vi "Main.vi"(11 "Module Admin":refnum<class "Delacor_lib_QMH_Module Admin.lvclass">) -> ()   [LabVIEW 2024, in "DQMH Power Requests.lvlib"]
doc: "This template is based off of the Queued Message Handler design pattern and the Queued Message Handler project template that ships with LabVIEW.\n\nThe main difference is that the queue is private to this module and communication between modules is performed via Broadcast and Request events.\n\nRequest events are wrapped in public API methods and are handled in the Event Handling Loop (EHL) of this VI. Any module can register for Broadcast events sent by this module. The EHL generates messages based on user interface actions.\n\nThe Message Handling Loop (MHL) processes messages generated by the EHL, or by other messages. The messages are string values, so new messages can be added easily to the Message Cases case structure in the MHL. Each message cluster can also provide an optional value for Message Data, which is a variant that can be converted to whatever message-specific data is required.\n_____\nBased on Delacor QMH Project Template 4.2.1.64.\n\n<b>Note:</b> This VI was modified by the <b>Validate DQMH Module</b> tool to have the module name be passed as the Additional Information parameter with an Error Reported broadcast.\n\n<b>Note:</b> This VI was modified by the <b>Validate DQMH Module</b> tool to call the Release Message Queue VI in the top-level Error case.\n\n<b>Note:</b> This VI was modified by the <b>Validate DQMH Module</b> tool to add a 'Panel Hidden' status updated broadcast to the Panel Close? event when External Launch = TRUE.\n\n<b>Note:</b> This VI was modified by the <b>Validate DQMH Module</b> tool to add a call to the Error Reported VI at the end of the 'Exit' MHL frame."
uses:
  DQMH Power Requests.lvlib
  <vilib>/Delacor/Delacor QMH/Libraries/Module Admin_class/Delacor_lib_QMH_Module Admin.lvclass
  Module Data--cluster.ctl
  <vilib>/Delacor/Delacor QMH/Libraries/Message Queue_class/Delacor_lib_QMH_Message Queue.lvclass/Delacor_lib_QMH_Message Queue.ctl
  Stop Argument--cluster.ctl
  <vilib>/Delacor/Delacor QMH/Libraries/Module Admin_class/Delacor_lib_QMH_Module Admin.lvclass/Delacor_lib_QMH_Module Admin.ctl
  Create Request Argument--cluster.ctl
  Create Request (Reply Payload)--cluster.ctl
  System Required Argument--cluster.ctl
  System Required (Reply Payload)--cluster.ctl
  Display Required Argument--cluster.ctl
  Display Required (Reply Payload)--cluster.ctl
  <vilib>/Utility/miscctls.llb/LVPointTypeDef.ctl
  <vilib>/Delacor/Delacor QMH/Libraries/Message Queue_class/Delacor_lib_QMH_Enqueue Message (Single).vi
  <vilib>/Delacor/Delacor QMH/Libraries/Module Admin_class/Delacor_lib_QMH_Get External Launch.vi
  <vilib>/Utility/error.llb/Error Cluster From Error Code.vi
  <vilib>/ErrorRing/Error Ring.xnode
  <vilib>/Delacor/Delacor QMH/Libraries/Message Queue_class/Delacor_lib_QMH_Message Queue.lvclass
panel:
  in  "Simulate MHL Error":bool
  in  "Simulate EHL Error":bool
  out "error out":errorcluster
  out "Status":string
  # "Other QMH Modules communicate with this Module via its Public API (wrappers for its Request Events).\n\nThis Module communicates with other Modules via its Broadcast Events.\nAny module that wants to get these messages, just registers for this module's Broadcast events."
  # "This template is for the Delacor Modified Queued Message Handler design pattern.\n\nSee the block diagram for more information on how to use this template."
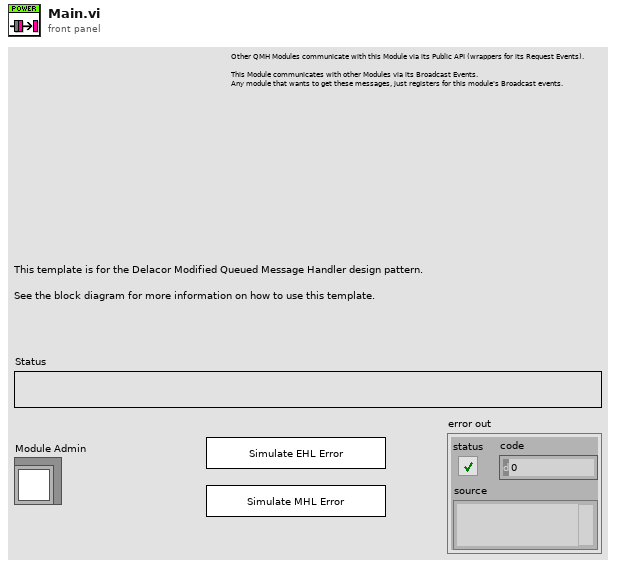
[diagram p1: front panel]
types:
  T1 = typedef "DQMH Power Requests.lvlib/Request Events--cluster.ctl" = cluster{"Stop Module":refnum<user-event>, "Show Panel":refnum<user-event>, "Hide Panel":refnum<user-event>, "Get Module Execution Status":refnum<user-event>, "Show Diagram":refnum<user-event>, "Create Request":refnum<user-event>, "System Required":refnum<user-event>, "Display Required":refnum<user-event>}
  T2 = typedef "DQMH Power Requests.lvlib/Module Data--cluster.ctl" = cluster{"Status":string, "Request Created":bool, "System Required":bool, "Display Required":bool}
  T3 = enum32{"invalid lock state", "Not Locked", "Locked (No Password)", "Password-protected"}
  T4 = typedef "DQMH Power Requests.lvlib/Stop Argument--cluster.ctl" = cluster{"Origin":string, "Exit via Stop Module Req?":bool, "Wait for Module to stop?":bool}
  T5 = typedef "DQMH Power Requests.lvlib/Create Request Argument--cluster.ctl" = cluster{"Simple Reason String":string, "Create":bool, "Wait Notifier":refnum<notifier>, "wait for reply":bool}
  T6 = typedef "DQMH Power Requests.lvlib/System Required Argument--cluster.ctl" = cluster{"Create":bool, "Wait Notifier":refnum<notifier>, "wait for reply":bool}
  T7 = typedef "DQMH Power Requests.lvlib/Display Required Argument--cluster.ctl" = cluster{"Create":bool, "Wait Notifier":refnum<notifier>, "wait for reply":bool}
  T8 = typedef "LVPointTypeDef.ctl" = cluster{"Horizontal":i16, "Vertical":i16}
  T9 = enum32{"Invalid", "Standard", "Closed", "Hidden", "Minimized", "Maximized"}
  T10 = typedef "DQMH Power Requests.lvlib/Create Request (Reply Payload)--cluster.ctl" = cluster{"Successful":bool, "Create Request_error":errorcluster}
  T11 = typedef "DQMH Power Requests.lvlib/System Required (Reply Payload)--cluster.ctl" = cluster{"Successful":bool, "System Required_error":errorcluster}
  T12 = typedef "DQMH Power Requests.lvlib/Display Required (Reply Payload)--cluster.ctl" = cluster{"Successful":bool, "Display Required_error":errorcluster}
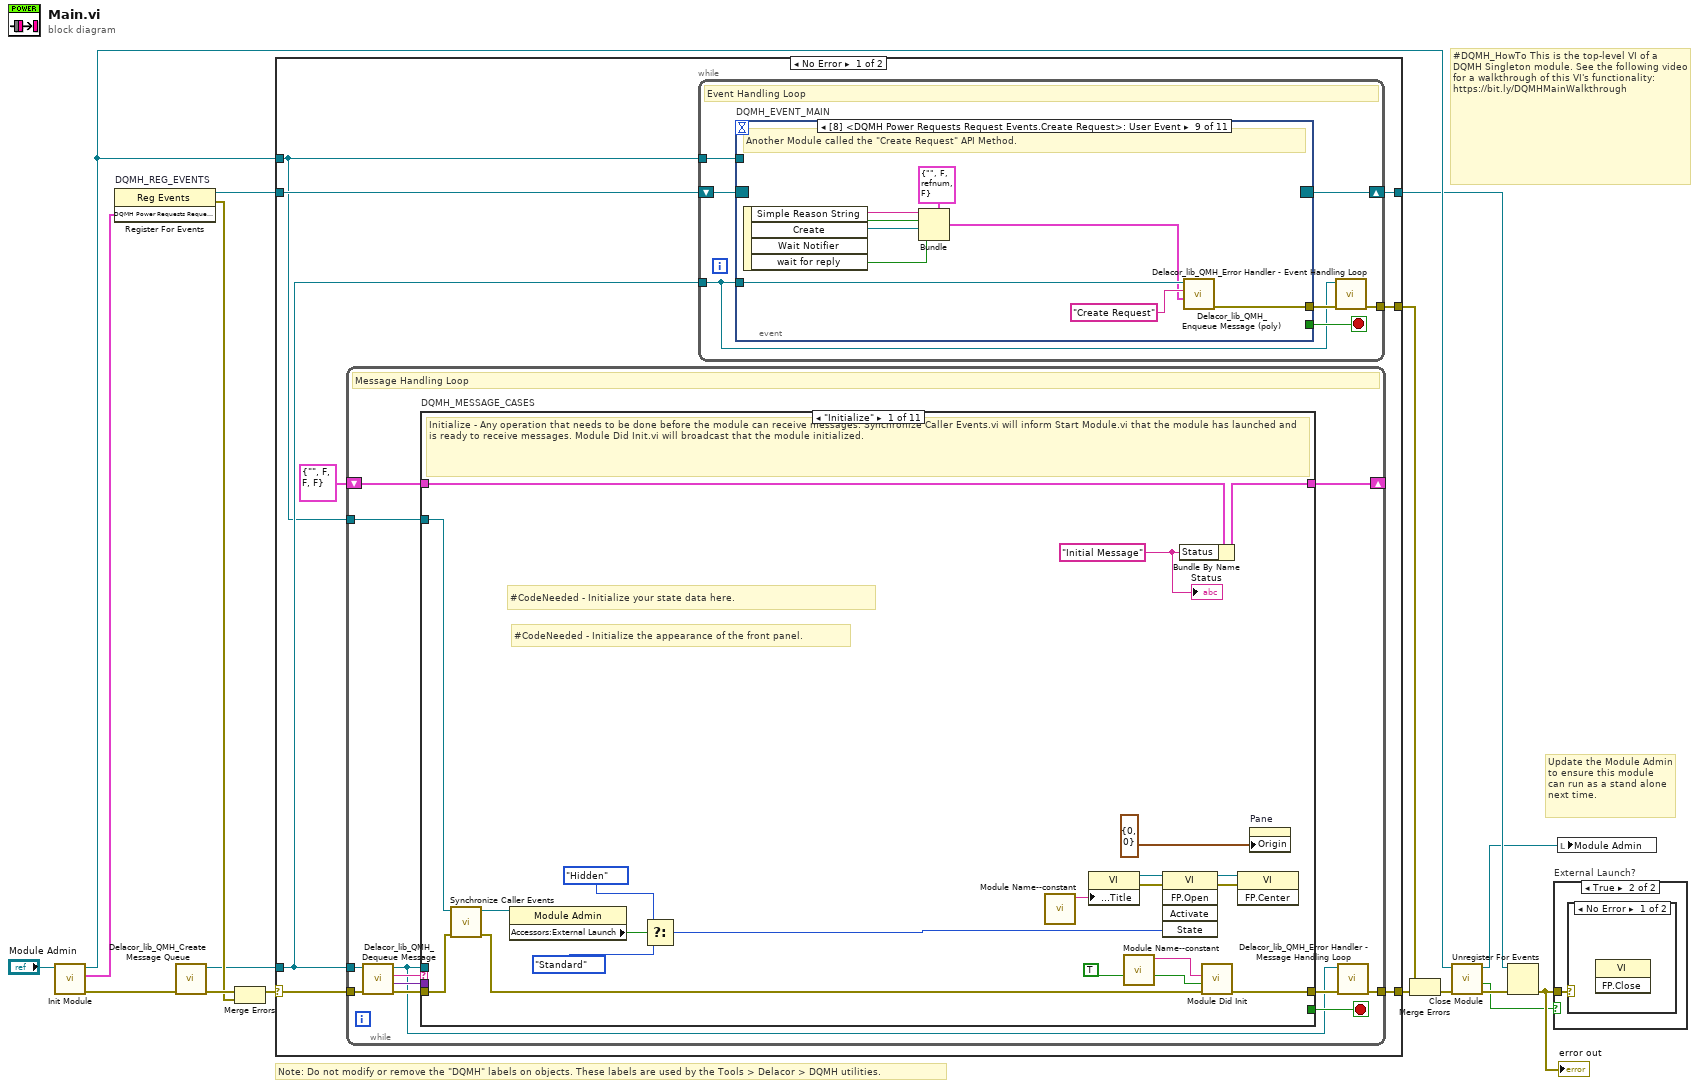
[diagram p0: block diagram]
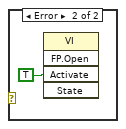
[diagram p3: hidden frame]
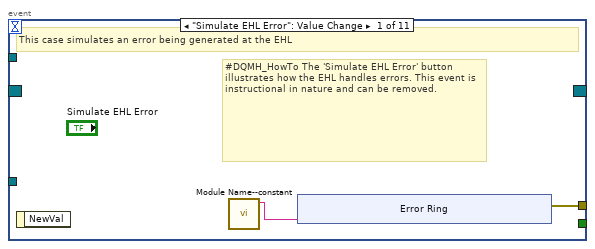
[diagram p4: hidden frame]
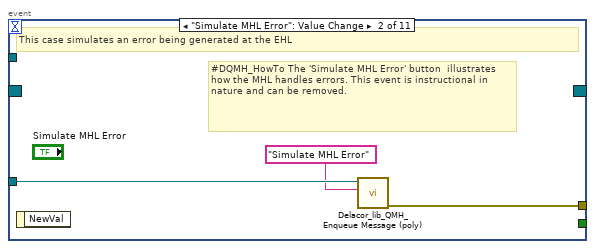
[diagram p5: hidden frame]
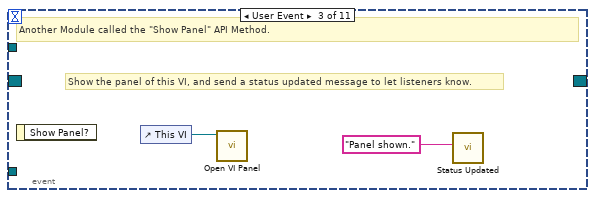
[diagram p6: hidden frame]
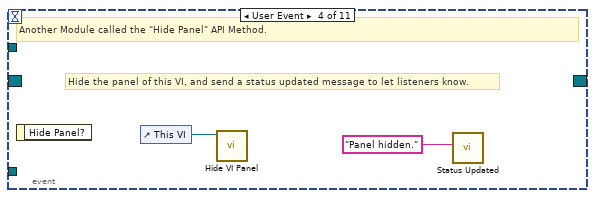
[diagram p7: hidden frame]
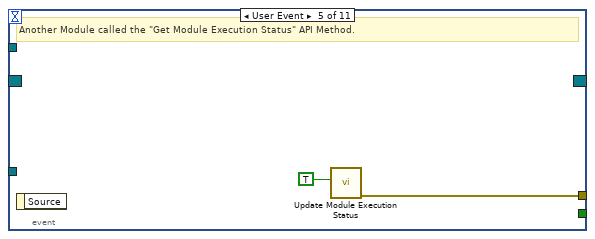
[diagram p8: hidden frame]
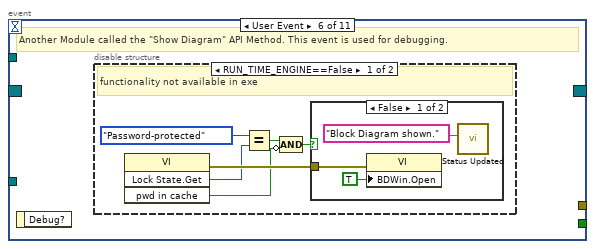
[diagram p9: hidden frame]
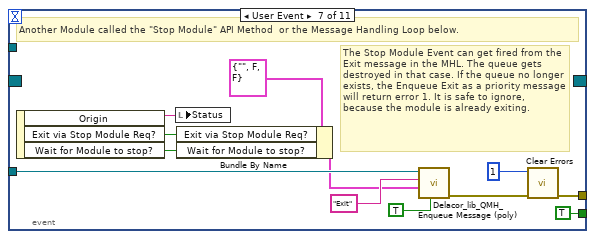
[diagram p12: hidden frame]
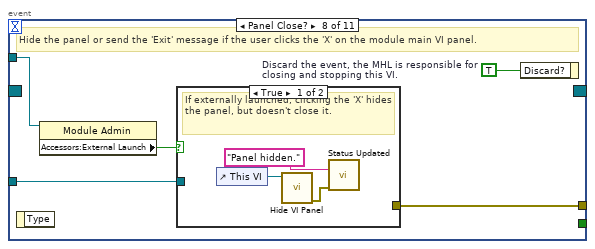
[diagram p13: hidden frame]
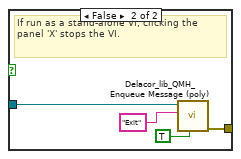
[diagram p14: hidden frame]
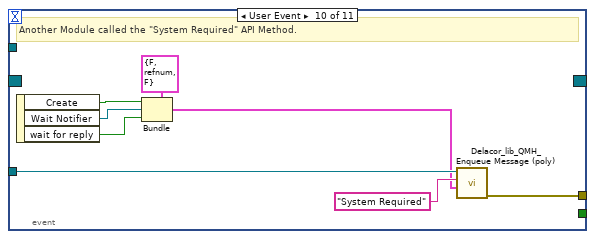
[diagram p15: hidden frame]
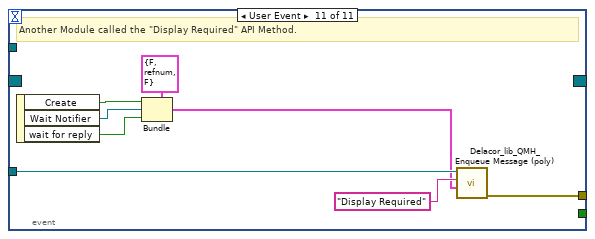
[diagram p16: hidden frame]
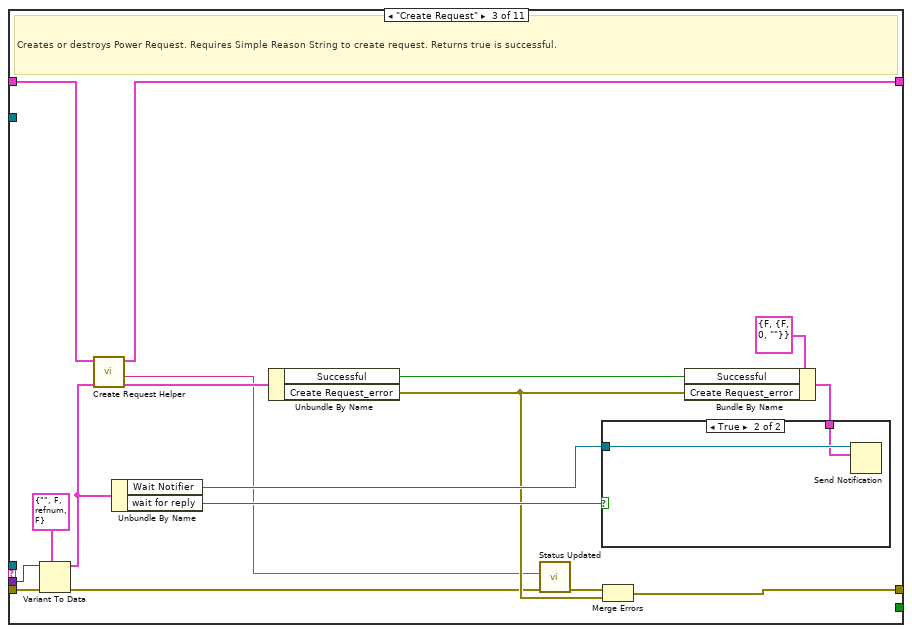
[diagram p18: hidden frame]
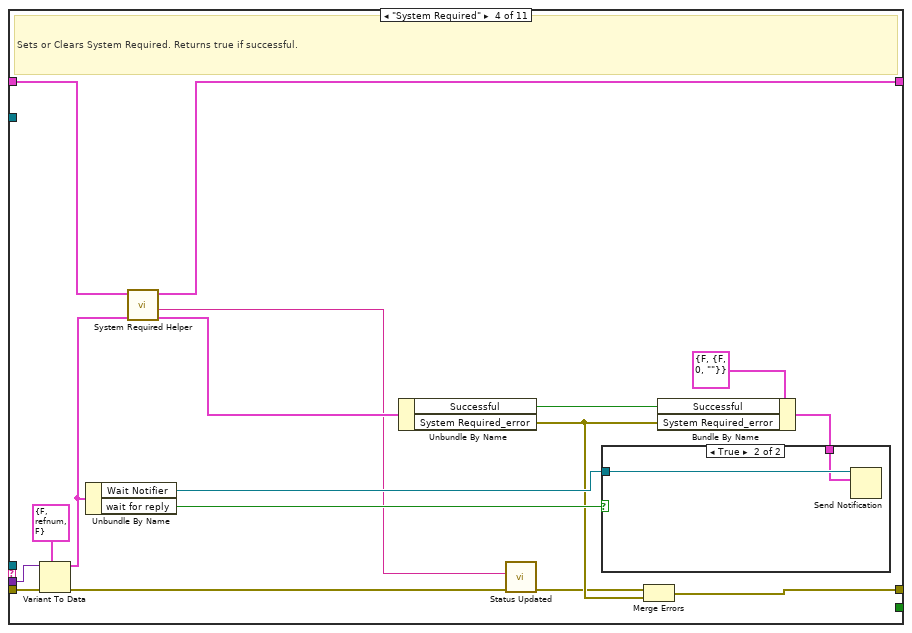
[diagram p20: hidden frame]
diagram:
  # "#DQMH_HowTo This is the top-level VI of a DQMH Singleton module. See the following video for a walkthrough of this VI's functionality: https://bit.ly/DQMHMainWalkthrough"
  # "Note: Do not modify or remove the \"DQMH\" labels on objects. These labels are used by the Tools > Delacor > DQMH utilities."
  # "Update the Module Admin to ensure this module can run as a stand alone next time."
  n1 = call "Init Module.vi"("Singleton Module Admin in"="Module Admin") -> ("error out"=w16:errorcluster, "DQMH Power Requests Request Events"=w5:T1, "Singleton Module Admin out"=w8:refnum<class "Delacor_lib_QMH_Module Admin.lvclass">)  [unwired: 8 in]
  n2 = register-events "DQMH_REG_EVENTS"(w5) -> (reference out=w6:refnum<event-registration>, error out=w9:errorcluster)  [unwired: 2 in]
  n3 = call <vilib>:"Delacor_lib_QMH_Create Message Queue.vi"("error in"=w16) -> ("error out"=w11:errorcluster, "Message Queue"=w4:refnum<class "Delacor_lib_QMH_Message Queue.lvclass">)  [unwired: 9 in]
  n4 = Merge Errors(w11, w9) -> (w10:errorcluster)
  n5 = case shown="No Error" w10 {
    selector: w10 -> [w23 w270]
    tunnel: [w25 w270] -> w17
    tunnel: [w22 w267] -> w7
    tunnel: w6 -> [w20 w267]
    tunnel: w4 -> [w19 w262]
    tunnel: [w24 _] -> w14
    tunnel: w8 -> [w18 w263]
    frame No Error {
      n6 = while {
        tunnel: w19 -> [w111]
        shift-right: [w115] -> _
        shift-left: T2 {"Status"="", "Request Created"=FALSE, "System Required"=FALSE, "Display Required"=FALSE} ("Data Cluster") -> [w116]
        tunnel: w23 -> [w119]
        tunnel: [w117] -> w25
        tunnel: w18 -> [w109]
        stop <- w114 stop-if-true
        # "Message Handling Loop"
        n7 = call-dynamic "Delacor_lib_QMH_Dequeue Message.vi"("error in"=w119, "Message Queue in"=w111) -> ("error out"=w118:errorcluster, "Message Data"=w112:variant, "Message"=w113:string, "Message Queue out"=w110:refnum<class "Delacor_lib_QMH_Message Queue.lvclass">)  [unwired: 6 in]
        n8 = case "DQMH_MESSAGE_CASES" shown="\"Initialize\"" w113 {
          selector: w113 -> [_ _ _ _ _ _ _ _ _ _ w249]
          tunnel: w110 -> [_ _ _ _ _ _ _ _ w219 w241 _]
          tunnel: w118 -> [w138 w142 w159 w178 w197 w202 w204 w209 w226 w247 w251]
          tunnel: [w136 w142 w152 w171 w190 w201 w204 w208 w222 w244 w252] -> w120
          tunnel: w116 -> [w127 w141 w151 w170 w189 w200 w203 w206 w221 w233 w250]
          tunnel: [w126 w141 w150 w169 w187 w200 w203 w206 w221 w233 w250] -> w115
          tunnel: [_ _ _ _ _ _ _ _ _ w240 _] -> w114
          tunnel: w112 -> [_ _ w158 w177 w196 _ _ _ w220 w239 _]
          tunnel: w109 -> [w128 _ _ _ _ _ _ _ w218 w234 _]
          frame "Initialize" {
            w121 = "Initial Message" ("Initial Message")
            # "#CodeNeeded - Initialize the appearance of the front panel."
            # "#CodeNeeded - Initialize your state data here."
            # "Initialize - Any operation that needs to be done before the module can receive messages. Synchronize Caller Events.vi will inform Start Module.vi that the module has launched and is ready to receive messages. Module Did Init.vi will broadcast that the module initialized."
            n9 = call "Synchronize Caller Events.vi"("error in (no error)"=w138, "Singleton Module Admin in"=w128) -> ("error out"=w137:errorcluster, "Singleton Module Admin out"=w123:refnum<class "Delacor_lib_QMH_Module Admin.lvclass">)  [unwired: 8 in]
            n10 = property class="Module Admin"(reference=w123) -> ("Accessors:External Launch"=w132:bool)  [unwired: 1 in, 2 out]
            n11 = Select(t=T9."Hidden" ("State"), s=w132, f=T9."Standard" ("State")) -> (s? t:f=w129:T9)
            n12 = call "Module Name--constant.vi"() -> ("Module Name"=w135:string)  [unwired: 11 in]
            n13 = property class="VI"("Front Panel.Title"=w135) -> (reference out=w134:refnum<vi>, error out=w140:errorcluster)  [unwired: 2 in]
            n14 = call "Module Name--constant.vi"() -> ("Module Name"=w124:string)  [unwired: 11 in]
            n15 = invoke class="VI" method="FP.Open"(reference=w134, error in=w140, "State"=w129) -> (reference out=w133:refnum<vi>, error out=w139:errorcluster)  [unwired: 2 in, 3 out]
            n16 = Bundle By Name(cluster=w127, "Status"=w121) -> (w126:T2)
            n17 = call "Module Did Init.vi"("error in (no error)"=w137, "Initialized?"=TRUE, "Origin"=w124) -> ("error out"=w136:errorcluster)  [unwired: 8 in]
            n18 = invoke class="VI" method="FP.Center"(reference=w133, error in=w139) -> ()  [unwired: 1 in, 3 out]
            n19 = property on="Pane" class="Pane"("Origin"=T8 {"Horizontal"=0, "Vertical"=0}) -> ()  [unwired: 2 in, 2 out]
            "Status" <- w121
          }
          frame "--- Module Specific ---" {
            # "Separator -- The following cases handle messages specific to this Module."
          }
          frame "Create Request" {
            # "Creates or destroys Power Request. Requires Simple Reason String to create request. Returns true is successful."
            n20 = Variant To Data(error in=w159, type=T5 {"Simple Reason String"="", "Create"=FALSE, "Wait Notifier"=refnum, "wait for reply"=FALSE} ("Create Request Argument"), Variant=w158) -> (data=w149:T5, error out=w145:errorcluster)
            n21 = call "Create Request Helper.vi"("Create Request Argument"=w149, "Module Data"=w151) -> ("Create Request (Reply Payload)"=w148:T10, "Message"=w143:string, "Module Data out"=w150:T2)  [unwired: 7 in]
            n22 = Unbundle By Name(w149) -> ("Wait Notifier"=w156:refnum<notifier>, "wait for reply"=w155:bool)
            n23 = Unbundle By Name(w148) -> ("Successful"=w147:bool, "Create Request_error"=w146:errorcluster)
            n24 = call "Status Updated.vi"("error in (no error)"=w145, "Status"=w143) -> ("error out"=w144:errorcluster)  [unwired: 9 in]
            n25 = Merge Errors(w144, w146) -> (w152:errorcluster)
            n26 = Bundle By Name(cluster=T10 {"Successful"=FALSE, "Create Request_error"={"status"=FALSE, "code"=0, "source"=""}} ("Create Request (Reply Payload)"), "Successful"=w147, "Create Request_error"=w146) -> (w154:T10)
            n27 = case shown="True" w155 {
              tunnel: w156 -> [_ w161]
              tunnel: w154 -> [_ w160]
              frame False {
              }
              frame True {
                n28 = Send Notification(notification=w160, notifier=w161) -> ()  [unwired: 1 in, 2 out]
              }
            }
          }
          frame "System Required" {
            # "Sets or Clears System Required. Returns true if successful."
            n29 = Variant To Data(error in=w178, type=T6 {"Create"=FALSE, "Wait Notifier"=refnum, "wait for reply"=FALSE} ("System Required Argument"), Variant=w177) -> (data=w168:T6, error out=w164:errorcluster)
            n30 = Unbundle By Name(w168) -> ("Wait Notifier"=w175:refnum<notifier>, "wait for reply"=w174:bool)
            n31 = call "System Required Helper.vi"("System Required Argument"=w168, "Module Data"=w170) -> ("System Required (Reply Payload)"=w167:T11, "Message"=w162:string, "Module Data out"=w169:T2)  [unwired: 7 in]
            n32 = Unbundle By Name(w167) -> ("Successful"=w166:bool, "System Required_error"=w165:errorcluster)
            n33 = call "Status Updated.vi"("error in (no error)"=w164, "Status"=w162) -> ("error out"=w163:errorcluster)  [unwired: 9 in]
            n34 = Merge Errors(w163, w165) -> (w171:errorcluster)
            n35 = Bundle By Name(cluster=T11 {"Successful"=FALSE, "System Required_error"={"status"=FALSE, "code"=0, "source"=""}} ("System Required (Reply Payload)"), "Successful"=w166, "System Required_error"=w165) -> (w173:T11)
            n36 = case shown="True" w174 {
              tunnel: w175 -> [_ w180]
              tunnel: w173 -> [_ w179]
              frame False {
              }
              frame True {
                n37 = Send Notification(notification=w179, notifier=w180) -> ()  [unwired: 1 in, 2 out]
              }
            }
          }
          frame "Display Required" {
            # "Sets or Clears Display Required. Returns true if successful."
            n38 = Variant To Data(error in=w197, type=T7 {"Create"=FALSE, "Wait Notifier"=refnum, "wait for reply"=FALSE} ("Display Required Argument"), Variant=w196) -> (data=w188:T7, error out=w183:errorcluster)
            n39 = Unbundle By Name(w188) -> ("Wait Notifier"=w194:refnum<notifier>, "wait for reply"=w193:bool)  [unwired: 1 out]
            n40 = call "Display Required Helper.vi"("Display Required Argument"=w188, "Module Data"=w189) -> ("Display Required (Reply Payload)"=w186:T12, "Message"=w181:string, "Module Data out"=w187:T2)  [unwired: 7 in]
            n41 = Unbundle By Name(w186) -> ("Successful"=w185:bool, "Display Required_error"=w184:errorcluster)
            n42 = call "Status Updated.vi"("error in (no error)"=w183, "Status"=w181) -> ("error out"=w182:errorcluster)  [unwired: 9 in]
            n43 = Bundle By Name(cluster=T12 {"Successful"=FALSE, "Display Required_error"={"status"=FALSE, "code"=0, "source"=""}} ("Display Required (Reply Payload)"), "Successful"=w185, "Display Required_error"=w184) -> (w192:T12)
            n44 = case shown="True" w193 {
              tunnel: w194 -> [_ w199]
              tunnel: w192 -> [_ w198]
              frame False {
              }
              frame True {
                n45 = Send Notification(notification=w198, notifier=w199) -> ()  [unwired: 1 in, 2 out]
              }
            }
            n46 = Merge Errors(w182, w184) -> (w190:errorcluster)
          }
          frame "---Copy This Frame---" {
            # "Duplicate this frame when creating new messages.  Change this comment in the duplicated frame to describe this message."
            n47 = Merge Errors(w202) -> (w201:errorcluster)
          }
          frame "--- Exit and Error Handling---" {
            # "Separator - The following cases handle errors and exit messages."
          }
          frame "Simulate MHL Error" {
            # "#DQMH_HowTo The 'Simulate MHL Error' button  illustrates how the MHL handles errors. This event is instructional in nature and can be removed."
            # "Simulate an error occurring at the MHL"
            n48 = call "Module Name--constant.vi"() -> ("Module Name"=w205:string)  [unwired: 11 in]
            n49 = xnode "Error Ring"("parameter 0"=w205) -> ("error out"=w207:errorcluster)
            n50 = Merge Errors(w209, w207) -> (w208:errorcluster)
          }
          frame "Error" {
            # "#CodeRecommended - If you ever change the name of this \"Error\" message, you'll need to update the name in the Check Loop Error.vi as well."
            # "#CodeRecommended - If the module is running in standalone mode (External Launch = FALSE), this code will pop up an error dialog and call the 'Exit' message if an error occurs. Add more fine-grained error handling here."
            # "Error - Check the error message data and respond accordingly. This message is sent by the \"Error Handler\" VIs at the end of each loop in this application."
            n51 = property class="Module Admin"(reference=w218) -> ("Accessors:External Launch"=w217:bool)  [unwired: 1 in, 2 out]
            n52 = Variant To Data(error in=w226, type=errorcluster {"status"=FALSE, "code"=0, "source"=""} ("error constant"), Variant=w220) -> (data=w227:errorcluster, error out=w224:errorcluster)
            n53 = call "Error Reported.vi"("Error"=w227) -> ()  [unwired: 10 in, 1 out]
            n54 = case shown="False" w217 {
              tunnel: [w232 _] -> w223
              tunnel: w219 -> [w230 _]
              tunnel: w227 -> [w231 _]
              frame False {
                # "If the module is running standalone, then pop up an error dialog and call the \"Exit\" message."
                n55 = call <vilib>:"Simple Error Handler.vi"("error in (no error)"=w231) -> ()  [unwired: 4 in, 5 out]
                n56 = call-poly <vilib>:"Delacor_lib_QMH_Enqueue Message (poly).vi"("Priority Message? (F)"=TRUE, "Message"="Exit", "Message Queue in"=w230) -> ("error out"=w232:errorcluster)  [unwired: 7 in, 1 out]
              }
              frame True {
                # "If the module was launched externally, calling the Error Reported broadcast VI is the only action performed by the \"Error\" message. The module's caller can then process the error appropriately."
              }
            }
            n57 = Merge Errors(w224, w223) -> (w222:errorcluster)
            n58 = local write "error out"(w222) -> ()
          }
          frame "Exit" {
            w238 = 91  # 91: not all Exit messages will have an argument
            w240 = TRUE  # Stop the VI
            # "Release the message queue reference"
            # "Exit - Exit the application."
            n59 = Variant To Data(error in=w247, type=T4 {"Origin"="", "Exit via Stop Module Req?"=FALSE, "Wait for Module to stop?"=FALSE} ("Stop Argument"), Variant=w239) -> (data=w236:T4, error out=w243:errorcluster)
            n60 = call <vilib>:"Clear Errors.vi"("error in (no error)"=w243, "specific error code to clear (0: all)"=w238) -> ("error out"=w246:errorcluster)  [unwired: 4 in, 1 out]
            n61 = call "Create Request Helper.vi"("Module Data"=w233) -> ()  [unwired: 8 in, 3 out]
            n62 = control-ref of="This VI"() -> (w235:refnum<vi>)
            n63 = call-dynamic "Delacor_lib_QMH_Release Message Queue.vi"("error in"=w246, "Message Queue"=w241) -> ("error out"=w245:errorcluster)  [unwired: 9 in]
            n64 = call "Handle Exit.vi"("Stop Argument"=w236, "Admin in"=w234, "VI reference"=w235) -> ("error out"=w242:errorcluster)  [unwired: 7 in, 1 out]
            n65 = Merge Errors(w245, w242) -> (w244:errorcluster)
            n66 = call "Error Reported.vi"("Error"=w244) -> ()  [unwired: 10 in, 1 out]
          }
          frame Default {
            # "'Default' case only runs if there is a message that isn't defined in any of the other cases.  Output a programming error."
            n67 = call "Module Name--constant.vi"() -> ("Module Name"=w248:string)  [unwired: 11 in]
            n68 = xnode "Error Ring"("parameter 0"=w249, "parameter 1"=w248) -> ("error out"=w253:errorcluster)
            n69 = Merge Errors(w251, w253) -> (w252:errorcluster)
          }
        }
        n70 = call-dynamic "Delacor_lib_QMH_Error Handler - Message Handling Loop.vi"("error in"=w120, "Message Queue in"=w110) -> ("dup error in"=w117:errorcluster)  [unwired: 8 in, 1 out]
      }
      n71 = while {
        tunnel: w19 -> [w26]
        shift-right: [w29] -> w22
        shift-left: w20 -> [w30]
        tunnel: [w31] -> w24
        tunnel: w18 -> [w27]
        stop <- w28 stop-if-true
        # "Event Handling Loop"
        n72 = event "DQMH_EVENT_MAIN" shown="[8] <DQMH Power Requests Request Events.Create Request>: User Event" {
          selector: w30 -> [_ _ _ _ _ _ _ _ _ _ _]
          dyn-events: [_ _ _ _ _ _ _ _ _ _ _] -> w29
          timeout: _ -> [_ _ _ _ _ _ _ _ _ _ _]
          tunnel: [_ _ _ _ _ _ TRUE ("Discard?") _ _ _ _] -> w28
          tunnel: w26 -> [_ w43 _ _ _ _ w67 w74 w92 w100 w108]
          tunnel: [w34 w44 _ _ w50 _ w70 w76 w84 w93 w101] -> w32
          tunnel: w27 -> [_ _ _ _ _ _ _ w73 _ _ _]
          event "Simulate EHL Error": Value Change {
            # "#DQMH_HowTo The 'Simulate EHL Error' button  illustrates how the EHL handles errors. This event is instructional in nature and can be removed."
            # "This case simulates an error being generated at the EHL"
            n73 = event-data() -> ()  [unwired: 1 in, 1 out]
            n74 = call "Module Name--constant.vi"() -> ("Module Name"=w33:string)  [unwired: 11 in]
            n75 = xnode "Error Ring"("parameter 0"=w33) -> ("error out"=w34:errorcluster)
          }
          event "Simulate MHL Error": Value Change {
            # "#DQMH_HowTo The 'Simulate MHL Error' button  illustrates how the MHL handles errors. This event is instructional in nature and can be removed."
            # "This case simulates an error being generated at the EHL"
            n76 = event-data() -> ()  [unwired: 1 in, 1 out]
            n77 = call-poly <vilib>:"Delacor_lib_QMH_Enqueue Message (poly).vi"("Message"="Simulate MHL Error", "Message Queue in"=w43) -> ("error out"=w44:errorcluster)  [unwired: 8 in, 1 out]
          }
          event User Event {
            # "Show the panel of this VI, and send a status updated message to let listeners know."
            # "Another Module called the \"Show Panel\" API Method."
            n78 = event-data() -> ()  [unwired: 1 in, 1 out]
            n79 = control-ref of="This VI"() -> (w46:refnum<vi>)
            n80 = call "Open VI Panel.vi"("VI"=w46) -> ()  [unwired: 10 in, 1 out]
            n81 = call "Status Updated.vi"("Status"="Panel shown." ("format string")) -> ()  [unwired: 10 in, 1 out]
          }
          event User Event {
            # "Hide the panel of this VI, and send a status updated message to let listeners know."
            # "Another Module called the \"Hide Panel\" API Method."
            n82 = event-data() -> ()  [unwired: 1 in, 1 out]
            n83 = control-ref of="This VI"() -> (w48:refnum<vi>)
            n84 = call "Hide VI Panel.vi"("VI"=w48) -> ()  [unwired: 10 in, 1 out]
            n85 = call "Status Updated.vi"("Status"="Panel hidden." ("format string")) -> ()  [unwired: 10 in, 1 out]
          }
          event User Event {
            # "Another Module called the \"Get Module Execution Status\" API Method."
            n86 = event-data() -> ()  [unwired: 1 in, 1 out]
            n87 = call "Update Module Execution Status.vi"("Running?"=TRUE) -> ("error out"=w50:errorcluster)  [unwired: 10 in]
          }
          event User Event {
            # "Another Module called the \"Show Diagram\" API Method. This event is used for debugging."
            n88 = event-data() -> ()  [unwired: 1 in, 1 out]
            n89 = disable-structure shown="RUN_TIME_ENGINE==False" {
              frame condition #0 (active) {
                # "functionality not available in exe"
                n90 = invoke class="VI" method="Lock State.Get"() -> (error out=w56:errorcluster, "Get Lock State"=w55:T3, "pwd in cache"=w52:bool)  [unwired: 4 in, 1 out]
                n91 = Equal?(x=T3."Password-protected", y=w55) -> (x = y?=w53:bool)
                n92 = Compound Arithmetic op=AND(w53, invert w52) -> (w51:bool)
                n93 = case shown="False" w51 {
                  tunnel: w56 -> [w59 _]
                  frame False {
                    n94 = property class="VI"(error in=w59, "BDWin.Open"=TRUE ("Block Diagram Window:Open")) -> ()  [unwired: 1 in, 2 out]
                    n95 = call "Status Updated.vi"("Status"="Block Diagram shown." ("format string")) -> ()  [unwired: 10 in, 1 out]
                  }
                  frame True {
                    # "Password-protected VI, and the password is not in the cache. Do not show the diagram."
                  }
                }
              }
              frame condition #1 {
              }
            }
          }
          event User Event {
            # "The Stop Module Event can get fired from the Exit message in the MHL. The queue gets destroyed in that case. If the queue no longer exists, the Enqueue Exit as a priority message will return error 1. It is safe to ignore, because the module is already exiting."
            # "Another Module called the \"Stop Module\" API Method  or the Message Handling Loop below."
            n96 = event-data() -> ("Origin"=w66:string, "Exit via Stop Module Req?"=w62:bool, "Wait for Module to stop?"=w61:bool)  [unwired: 1 in]
            n97 = local write "Status"(w66) -> ()
            n98 = Bundle By Name(cluster=T4 {"Origin"="", "Exit via Stop Module Req?"=FALSE, "Wait for Module to stop?"=FALSE} ("Stop Argument"), "Exit via Stop Module Req?"=w62, "Wait for Module to stop?"=w61) -> (w60:T4)
            n99 = call-poly <vilib>:"Delacor_lib_QMH_Enqueue Message (poly).vi"("Priority Message? (F)"=TRUE, "Message Data"=w60, "Message"="Exit", "Message Queue in"=w67) -> ("error out"=w71:errorcluster)  [unwired: 6 in, 1 out]
            n100 = call <vilib>:"Clear Errors.vi"("error in (no error)"=w71, "specific error code to clear (0: all)"=1) -> ("error out"=w70:errorcluster)  [unwired: 4 in, 1 out]
          }
          event Panel Close? {
            w75 = TRUE  # Discard the event, the MHL is responsible for closing and stopping this VI.
            # "Hide the panel or send the 'Exit' message if the user clicks the 'X' on the module main VI panel."
            n101 = event-data() -> ()  [unwired: 1 in, 1 out]
            n102 = property class="Module Admin"(reference=w73) -> ("Accessors:External Launch"=w72:bool)  [unwired: 1 in, 2 out]
            n103 = case shown="True" w72 {
              tunnel: w74 -> [_ w82]
              tunnel: [_ w83] -> w76
              frame True {
                # "If externally launched, clicking the 'X' hides the panel, but doesn't close it."
                n104 = control-ref of="This VI"() -> (w79:refnum<vi>)
                n105 = call "Hide VI Panel.vi"("VI"=w79) -> ("error out"=w77:errorcluster)  [unwired: 10 in]
                n106 = call "Status Updated.vi"("error in (no error)"=w77, "Status"="Panel hidden.") -> ()  [unwired: 9 in, 1 out]
              }
              frame False {
                # "If run as a stand-alone VI, clicking the panel 'X' stops the VI."
                n107 = call-poly <vilib>:"Delacor_lib_QMH_Enqueue Message (poly).vi"("Priority Message? (F)"=TRUE, "Message"="Exit", "Message Queue in"=w82) -> ("error out"=w83:errorcluster)  [unwired: 7 in, 1 out]
              }
            }
            n108 = event-data("Discard?"=w75) -> ()  [unwired: 1 in, 1 out]
          }
          event User Event {
            # "Another Module called the \"Create Request\" API Method."
            n109 = event-data() -> ("Simple Reason String"=w88:string, "Create"=w87:bool, "Wait Notifier"=w86:refnum<notifier>, "wait for reply"=w85:bool)  [unwired: 1 in]
            n110 = Bundle(cluster=T5 {"Simple Reason String"="", "Create"=FALSE, "Wait Notifier"=refnum, "wait for reply"=FALSE} ("Create Request Argument"), "Simple Reason String"=w88, "Create"=w87, "Wait Notifier"=w86, "wait for reply"=w85) -> (w89:T5)
            n111 = call-poly <vilib>:"Delacor_lib_QMH_Enqueue Message (poly).vi"("Message Data"=w89, "Message"="Create Request", "Message Queue in"=w92) -> ("error out"=w84:errorcluster)  [unwired: 7 in, 1 out]
          }
          event User Event {
            # "Another Module called the \"System Required\" API Method."
            n112 = event-data() -> ("Create"=w96:bool, "Wait Notifier"=w95:refnum<notifier>, "wait for reply"=w94:bool)  [unwired: 1 in]
            n113 = Bundle(cluster=T6 {"Create"=FALSE, "Wait Notifier"=refnum, "wait for reply"=FALSE} ("System Required Argument"), "Create"=w96, "Wait Notifier"=w95, "wait for reply"=w94) -> (w97:T6)
            n114 = call-poly <vilib>:"Delacor_lib_QMH_Enqueue Message (poly).vi"("Message Data"=w97, "Message"="System Required", "Message Queue in"=w100) -> ("error out"=w93:errorcluster)  [unwired: 7 in, 1 out]
          }
          event User Event {
            # "Another Module called the \"Display Required\" API Method."
            n115 = event-data() -> ("Create"=w104:bool, "Wait Notifier"=w103:refnum<notifier>, "wait for reply"=w102:bool)  [unwired: 1 in]
            n116 = Bundle(cluster=T7 {"Create"=FALSE, "Wait Notifier"=refnum, "wait for reply"=FALSE} ("Display Required Argument"), "Create"=w104, "Wait Notifier"=w103, "wait for reply"=w102) -> (w105:T7)
            n117 = call-poly <vilib>:"Delacor_lib_QMH_Enqueue Message (poly).vi"("Message Data"=w105, "Message"="Display Required", "Message Queue in"=w108) -> ("error out"=w101:errorcluster)  [unwired: 7 in, 1 out]
          }
        }
        n118 = call-dynamic "Delacor_lib_QMH_Error Handler - Event Handling Loop.vi"("error in"=w32, "Message Queue in"=w26) -> ("dup error in"=w31:errorcluster)  [unwired: 8 in, 1 out]
      }
    }
    frame Error {
      # "Synchronize Caller Events.vi will inform Start Module.vi that the module has launched and will let the code calling Start Module.vi register for broadcasts and would permit the caller receive the broadcast that an error occurred at launch time."
      n119 = call "Synchronize Caller Events.vi"("Singleton Module Admin in"=w263) -> ("error out"=w268:errorcluster)  [unwired: 9 in, 1 out]
      n120 = call-dynamic "Delacor_lib_QMH_Release Message Queue.vi"("Message Queue"=w262) -> ()  [unwired: 10 in, 1 out]
      n121 = call "Module Name--constant.vi"() -> ("Module Name"=w266:string)  [unwired: 11 in]
      n122 = Format Into String(format string="An error occurred during initialization. %s is no longer running.", w266) -> (resulting string=w264:string)  [unwired: 2 in, 1 out]
      n123 = Merge Errors(w270, w268) -> (w269:errorcluster)
      n124 = call "Error Reported.vi"("Additional Information"=w264, "Error"=w269) -> ()  [unwired: 9 in, 1 out]
    }
  }
  n125 = Merge Errors(w14, w17) -> (w13:errorcluster)
  n126 = call "Close Module.vi"("error in (no error)"=w13, "Module Admin in"=w8) -> ("error out"=w15:errorcluster, "External Launch"=w1:bool, "Module Admin out"=w2:refnum<class "Delacor_lib_QMH_Module Admin.lvclass">)  [unwired: 7 in]
  n127 = Unregister For Events(event registration refnum=w7, error in=w15) -> (error out=w12:errorcluster)
  "error out" <- w12
  n128 = case "External Launch?" shown="True" w1 {
    tunnel: w12 -> [_ w271]
    frame False {
    }
    frame True {
      n129 = case shown="No Error" w271 {
        frame No Error {
          n130 = invoke class="VI" method="FP.Close"() -> ()  [unwired: 3 in, 3 out]
        }
        frame Error {
          n131 = invoke class="VI" method="FP.Open"("Activate"=TRUE ("Activate?")) -> ()  [unwired: 4 in, 5 out]
        }
      }
    }
  }
  n132 = local write "Module Admin"(w2) -> ()
